vi "calcAddressInMemory(divider4).vi"(0 "Width":u16, 1 "Rows":u16, 3 "delayRowCount":u8, 5 "Cols":u16) -> (7 "addressInMemory":u16)   [LabVIEW 2016]
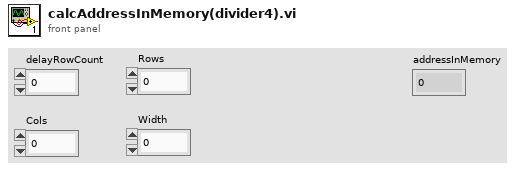
[diagram p1: front panel]
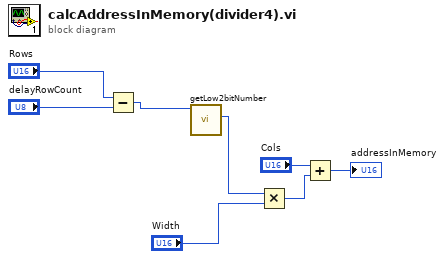
[diagram p0: block diagram]
diagram:
  n1 = Subtract(x="Rows", y="delayRowCount") -> (x-y=w2:u16)
  n2 = call "getLow2bitNumber.vi"("number"=w2) -> ("outputNum"=w1:u8)  [unwired: 10 in]
  n3 = Multiply(x=w1, y="Width") -> (x*y=w5:u16)
  n4 = Add(x="Cols", y=w5) -> (x+y=→"addressInMemory":u16)
